vi "test image click.vi"() -> ()   [LabVIEW 2010]
uses:
  <vilib>/Utility/miscctls.llb/LVPoint32TypeDef.ctl
panel:
  out "x-y":cluster{u32, u32}
  in  "stop":bool
  out "Coordinates":i32[](array[numeric])
  out "Coords":T1
  out "test image":T2(plugin-control)
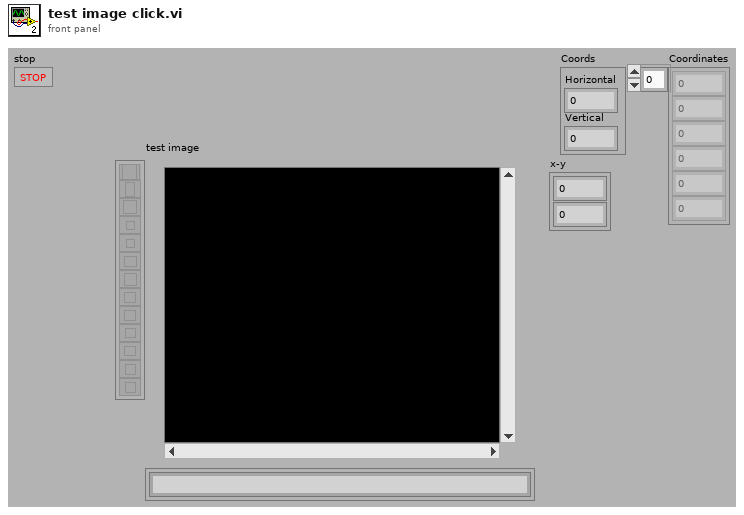
[diagram p1: front panel]
types:
  T1 = typedef "LVPoint32TypeDef.ctl" = cluster{"Horizontal":i32, "Vertical":i32}
  T2 = typedef "IMAQ Image.ctl" = refnum<image>
  T3 = typedef "Image Type" = u32
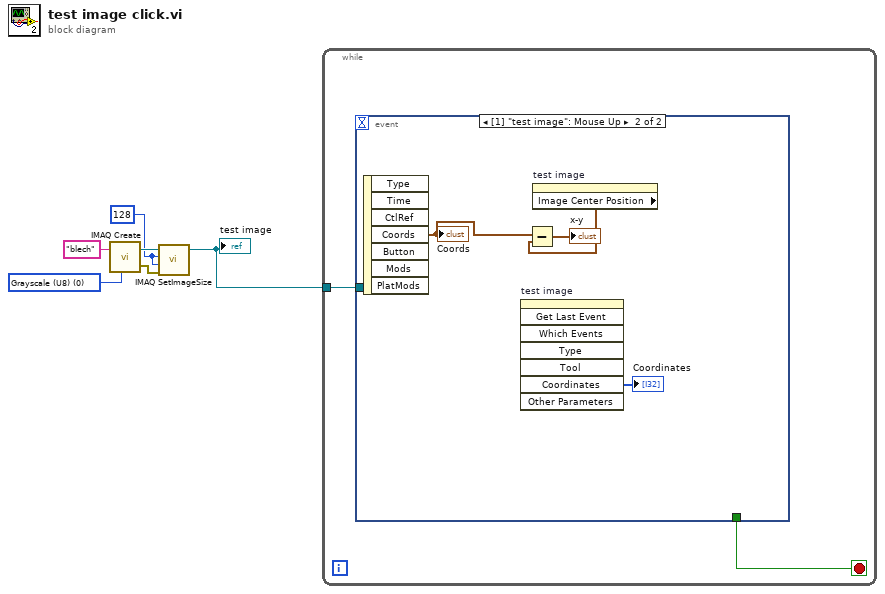
[diagram p0: block diagram]
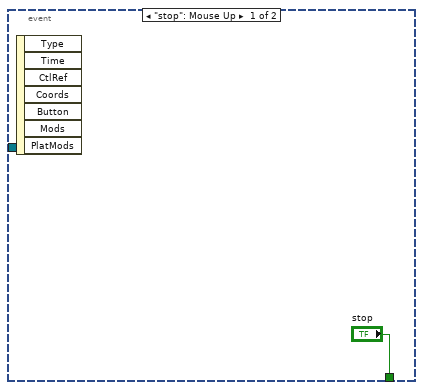
[diagram p2: hidden frame]
diagram:
  w2 = 128 ("X Resolution")
  w5 = T3 0 items=["Grayscale (U8)", "Grayscale (I16)", "Grayscale (SGL)", "Complex (CSG)", "RGB (U32)", "HSL (U32)", "RGB (U64)", "Grayscale (U16)"] ("Image Type")
  n1 = call "IMAQ Create"("Image Name"="blech", "Image Type"=w5) -> ("New Image"=w4:T2, "error out"=w3:errorcluster)  [unwired: 3 in]
  n2 = call "IMAQ SetImageSize"("error in (no error)"=w3, "Y Resolution"=w2, "X Resolution"=w2, "Image"=w4) -> ("Image Out"=w1:T2)  [unwired: 1 in, 1 out]
  "test image" <- w1
  n3 = while {
    tunnel: w1 -> [w8]
    stop <- w7 stop-if-true
    n4 = event shown="[1] \"test image\": Mouse Up" {
      selector: _ -> [_ _]
      dyn-events: _ -> [_ _]
      timeout: _ -> [_ _]
      tunnel: w8 -> [_ _]
      tunnel: ["stop" _] -> w7
      event "stop": Mouse Up {
        n5 = event-data() -> ()  [unwired: 1 in, 7 out]
      }
      event "test image": Mouse Up {
        n6 = event-data() -> ("Coords"=w12:T1)  [unwired: 1 in, 6 out]
        "Coords" <- w12
        n7 = invoke on="test image" class="ImageControl" method="Get Last Event"() -> ("Coordinates"=→"Coordinates":i32[])  [unwired: 8 in, 7 out]
        n8 = property on="test image" class="ImageControl"() -> ("Image Center Position"=w11:cluster{"X":u32, "Y":u32})  [unwired: 2 in, 2 out]
        n9 = Subtract(x=w12, y=w11) -> (x-y=→"x-y":cluster{u32, u32})
      }
    }
  }
